vi "GaussianKernel.vi"() -> ()   [LabVIEW 2017]
uses:
  <vilib>/Analysis/Matrix/Datatypes/RealMatrix.ctl
  <vilib>/vision/NI_Vision_Development_Module.lvlib
  <vilib>/Analysis/Matrix/NI_Matrix.lvlib
panel:
  out "Kernel":T1
  out "Image":T2(plugin-control)
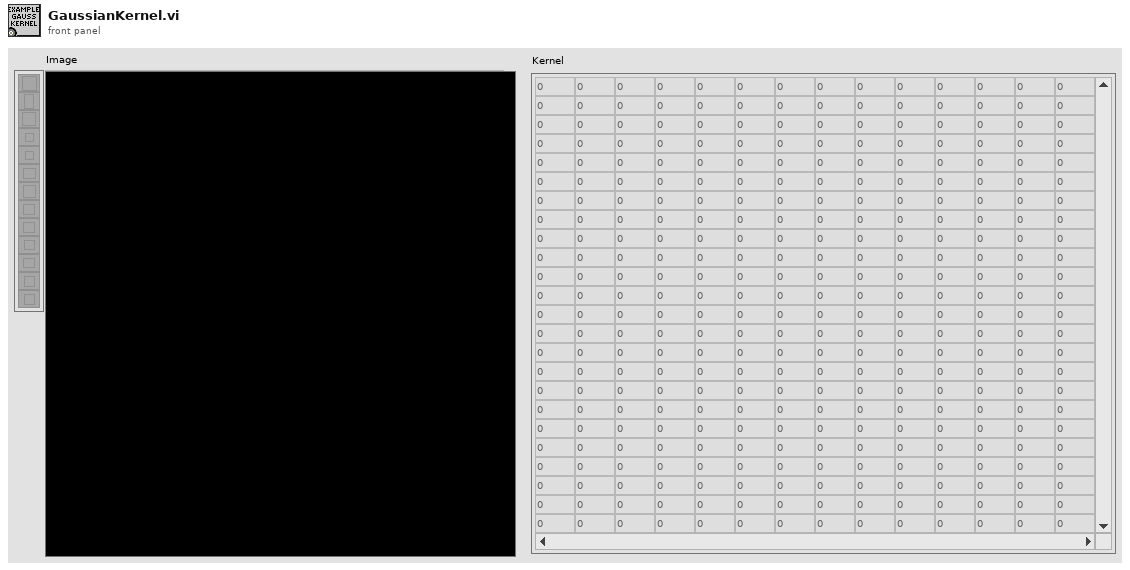
[diagram p1: front panel]
types:
  T1 = typedef "NI_Matrix.lvlib/RealMatrix.ctl" = dbl[][]
  T2 = typedef "IMAQ Image.ctl" = refnum<image>
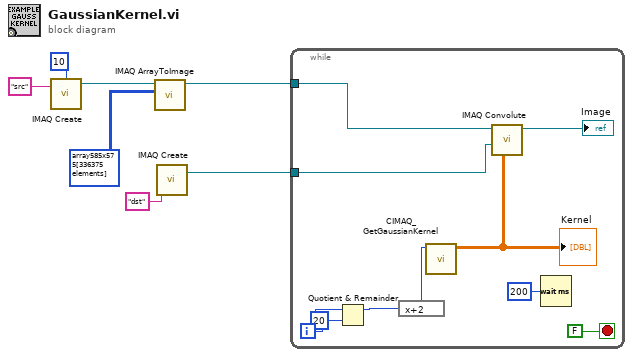
[diagram p0: block diagram]
diagram:
  n1 = call "IMAQ Create"("Border Size"=10, "Image Name"="src") -> ("New Image"=w3:T2)  [unwired: 3 in, 1 out]
  n2 = call "IMAQ ArrayToImage"("Image Pixels (U8)"=u8[][] array585x575[336375 elements] ("Image Pixels (U8) 2"), "Image"=w3) -> ("Image Out"=w2:T2)  [unwired: 8 in, 1 out]
  n3 = call "IMAQ Create"("Image Name"="dst") -> ("New Image"=w5:T2)  [unwired: 4 in, 1 out]
  n4 = while {
    tunnel: w2 -> [w13]
    tunnel: w5 -> [w11]
    i -> [w16]
    stop <- FALSE stop-if-true
    n5 = Quotient & Remainder(x=w16, y=20) -> (x-y*floor(x/y)=w14:i32)  [unwired: 1 out]
    n6 = expression code="x+2"(w14) -> (w8:i32)
    n7 = call <userlib>:"CIMAQ_GetGaussianKernel.vi"("Size"=w8) -> ("Kernel"=w12:T1)  [unwired: 10 in]
    "Kernel" <- w12
    n8 = call "IMAQ Convolute"("Kernel"=w12, "Image Dst"=w11, "Image Src"=w13) -> ("Image Dst Out"=→"Image":T2)  [unwired: 7 in, 1 out]
    n9 = Wait (ms)(milliseconds to wait=u32 200) -> ()  [unwired: 1 out]
  }
